vi "Calculator.vi"() -> ()   [LabVIEW 2019]
panel:
  in  "stop":bool
  out "Hasil":dbl
  in  "Operation":enum16{"+", "-", "/", "*"}(ring)
  in  "Angka 2":dbl
  in  "Angka 1":dbl
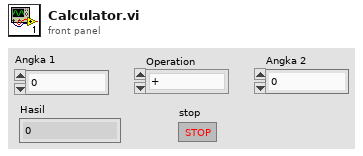
[diagram p1: front panel]
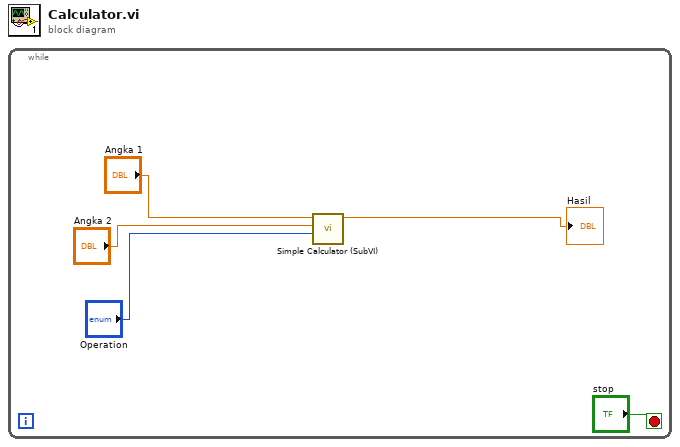
[diagram p0: block diagram]
diagram:
  n1 = while {
    stop <- "stop" stop-if-true
    n2 = call "Simple Calculator (SubVI).vi"("Operation"="Operation", "Angka in"="Angka 2", "Angka 1"="Angka 1") -> ("Hasil"=→"Hasil":dbl)  [unwired: 8 in]
  }
